vi "Self Test.vi"(8 "error in":errorcluster, 10 "Board Image":T2, 11 "Component in":refnum<class "Component.lvclass">) -> (0 "error out":errorcluster, 2 "Pass?":T1, 3 "Component out":refnum<class "Component.lvclass">)   [LabVIEW 2023, in "Component.lvclass"]
doc: "Check the image for this component's placement on the board."
uses:
  Component.lvclass
  Common/Board Image.ctl
  Common/Pass Fail Boolean.ctl
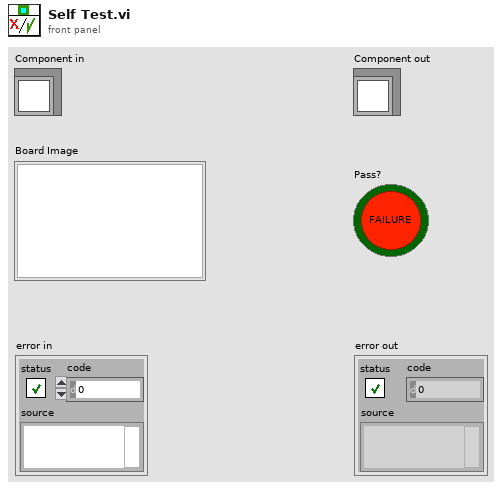
[diagram p1: front panel]
types:
  T1 = typedef "Pass Fail Boolean.ctl" = bool
  T2 = typedef "Board Image.ctl" = picture
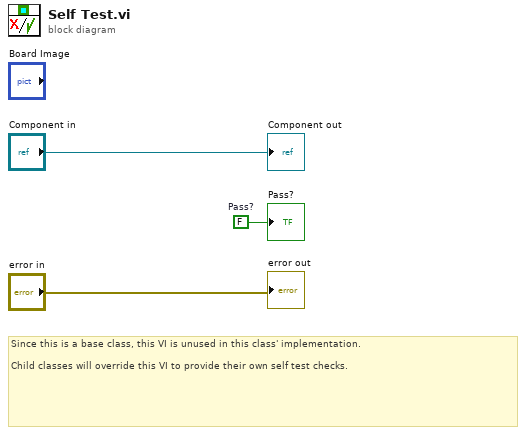
[diagram p0: block diagram]
diagram:
  w1 = T1 FALSE  # Pass?
  # "Since this is a base class, this VI is unused in this class' implementation.\n\nChild classes will override this VI to provide their own self test checks."
  "error out" <- "error in"
  "Component out" <- "Component in"
  "Pass?" <- w1
